vi "Read INI File (Gen).vi"(8 "error in":errorcluster, 11 "Path":path) -> (0 "error out":errorcluster, 1 "Scaling Coefficients":T1, 2 "DER_Info":T4, 3 "Generator_Info":T6)   [LabVIEW 2018]
uses:
  <vilib>/ORNL/CSEISMIC DDS/CSEISMIC DDS Base/Data Types/Generator_Info.ctl
  <vilib>/ORNL/CSEISMIC DDS/CSEISMIC DDS Base/Data Types/Controls/DeviceID.ctl
  <vilib>/ORNL/CSEISMIC DDS/CSEISMIC DDS Base/Data Types/Controls/EfficiencyCurve.ctl
  <vilib>/ORNL/CSEISMIC DDS/CSEISMIC DDS Base/Data Types/DER_Info.ctl
  Controls/Scaling Coefficients Cluster.ctl
  Controls/Scaling Coefficients Measurements.ctl
  Controls/Scaling Coefficients Setpoints.ctl
  <vilib>/Utility/config.llb/NI_LVConfig.lvlib
  <vilib>/ORNL/CSEISMIC DDS/CSEISMIC DDS Base/CSEISMIC DDS.lvclass
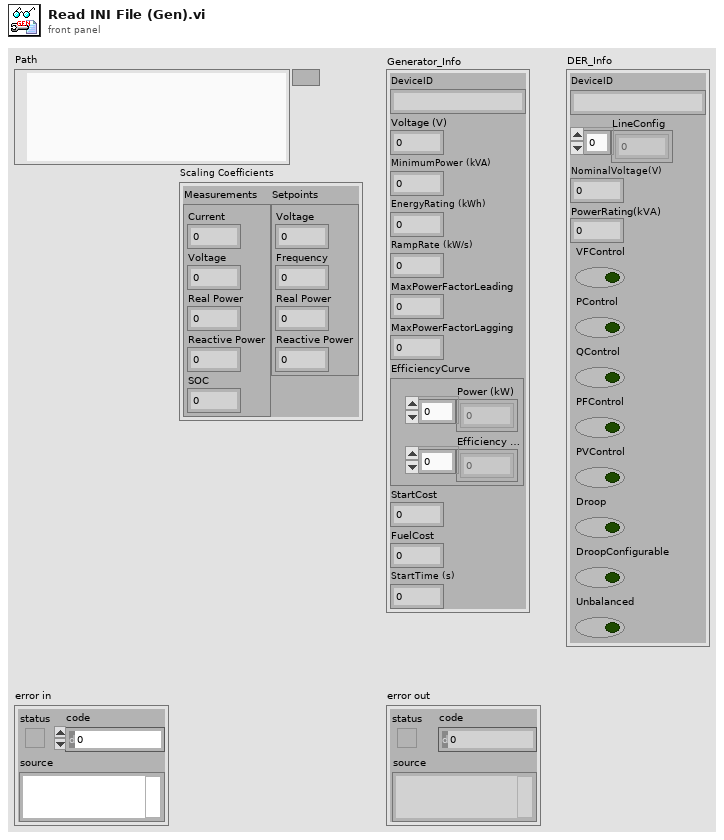
[diagram p1: front panel]
types:
  T1 = typedef "Scaling Coefficients Cluster.ctl" = cluster{"Measurements":T2, "Setpoints":T3}
  T2 = typedef "Scaling Coefficients Measurements.ctl" = cluster{"Current":dbl, "Voltage":dbl, "Real Power":dbl, "Reactive Power":dbl, "SOC":dbl}
  T3 = typedef "Scaling Coefficients Setpoints.ctl" = cluster{"Voltage":dbl, "Frequency":dbl, "Real Power":dbl, "Reactive Power":dbl}
  T4 = typedef "CSEISMIC DDS.lvlib/CSEISMIC DDS.lvclass/DER_Info.ctl" = cluster{"DeviceID":T5, "LineConfig":u8[], "NominalVoltage(V)":dbl, "PowerRating(kVA)":dbl, "VFControl":bool, "PControl":bool, "QControl":bool, "PFControl":bool, "PVControl":bool, "Droop":bool, "DroopConfigurable":bool, "Unbalanced":bool}
  T5 = typedef "CSEISMIC DDS.lvlib/CSEISMIC DDS.lvclass/DeviceID.ctl" = string
  T6 = typedef "CSEISMIC DDS.lvlib/CSEISMIC DDS.lvclass/Generator_Info.ctl" = cluster{"DeviceID":T5, "Voltage (V)":dbl, "MinimumPower (kVA)":dbl, "EnergyRating (kWh)":dbl, "RampRate (kW/s)":dbl, "MaxPowerFactorLeading":dbl, "MaxPowerFactorLagging":dbl, "EfficiencyCurve":T7, "StartCost":dbl, "FuelCost":dbl, "StartTime (s)":dbl}
  T7 = typedef "CSEISMIC DDS.lvlib/CSEISMIC DDS.lvclass/EfficiencyCurve.ctl" = cluster{"Power (kW)":dbl[], "Efficiency (%)":dbl[]}
  T8 = typedef "NI_LVConfig.lvlib/Config Data RefNum.ctl" = refnum<k1>
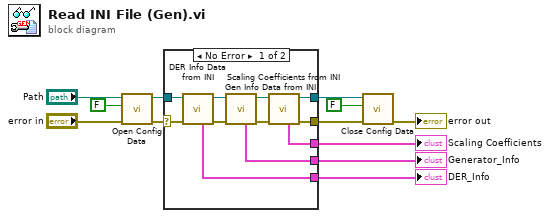
[diagram p0: block diagram]
diagram:
  n1 = call <vilib>:"Open Config Data.vi"("error in (no error)"="error in", "create file if necessary (T)"=FALSE, "configuration file path"="Path") -> ("error out"=w10:errorcluster, "refnum"=w9:T8)  [unwired: 6 in, 1 out]
  n2 = case shown="No Error" w10 {
    selector: w10 -> [w22 w24]
    tunnel: w9 -> [w23 w25]
    tunnel: [w19 _] -> w5
    tunnel: [w18 _] -> w4
    tunnel: [w16 w25] -> w8
    tunnel: [w14 w24] -> w7
    tunnel: [w13 _] -> w1
    frame No Error {
      n3 = call "DER Info Data from INI.vi"("error in"=w22, "Config Refnum in"=w23) -> ("error out"=w20:errorcluster, "Config Refnum out"=w21:T8, "DER_Info"=w18:T4)  [unwired: 7 in]
      n4 = call "Gen Info Data from INI.vi"("error in"=w20, "Config Refnum in"=w21) -> ("error out"=w15:errorcluster, "Config Refnum out"=w17:T8, "Generator_Info"=w19:T6)  [unwired: 7 in]
      n5 = call "Scaling Coefficients from INI.vi"("error in"=w15, "Config Refnum in"=w17) -> ("error out"=w14:errorcluster, "Config Refnum out"=w16:T8, "Scaling Coefficients"=w13:T1)  [unwired: 7 in]
    }
    frame Error {
    }
  }
  "Generator_Info" <- w5
  "DER_Info" <- w4
  "Scaling Coefficients" <- w1
  n6 = call <vilib>:"Close Config Data.vi"("error in (no error)"=w7, "write file if changed (T)"=FALSE, "refnum"=w8) -> ("error out"=→"error out":errorcluster)  [unwired: 7 in, 1 out]
